vi "Get_ADAM_averages_server.vi"(5 "No of averages":i32=1, 6 "All Active Channels":bool, 7 "End time":dbl, 8 "Start time":dbl, 9 "Clients time":dbl, 10 "ADAM Ch Names":string[](array[string])) -> (0 "DBL values":dbl[][](array[numeric]) format="%.2f", 1 "Values":string[][](array[string]), 2 "Comments":string[](array[string]), 3 "Titles":string[](array[string]), 4 "Times":dbl[](array[numeric]) format="%.2f")   [LabVIEW 2021]
uses:
  ADAM_Global.vi
  Sub VI's/Logged_Data_real_Global.vi
  Sub VI's/Channel_Description_Global.vi
panel:
  out "Client leads me by:":dbl
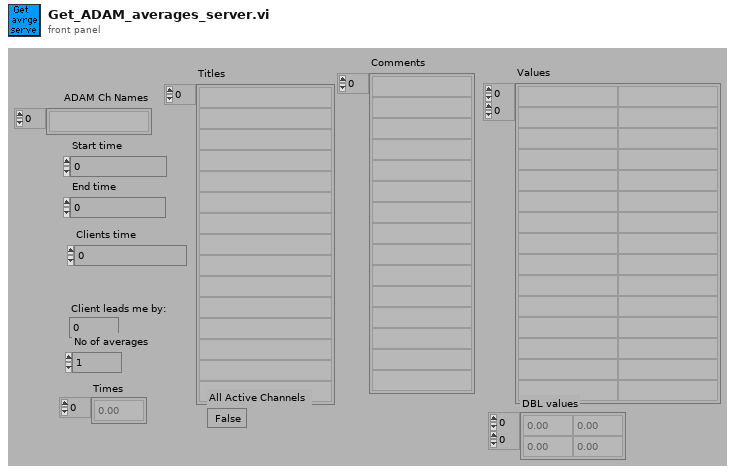
[diagram p1: front panel]
types:
  T1 = typedef "Update_scan_value.ctl" = cluster{"Channel Name":string, "New Value":dbl, "!Auto_Off":bool}
  T2 = typedef "Ch_description_ADAM.ctl" = cluster{"Ch Name":string, "Type":T3, "Function":T4, "Ch State":T5, "Calibration type":T6, "A":dbl, "B":dbl, "C":dbl, "D":dbl, "Comments":string, "Address":T7, "String":string, "Duty":u16}
  T3 = typedef "Module_type_ADAM.ctl" = string
  T4 = typedef "Function_ADAM.ctl" = enum16{"Analogue Input", "Digital Input", "Event counter", "Event rate", "Analogue Output", "Digital Output", "Relay Output"}
  T5 = typedef "Channel_State.ctl" = enum16{"On", "Off", "Always On", "Always Off"}
  T6 = typedef "Calib_type_ADAM.ctl" = string
  T7 = typedef "Address.ctl" = cluster{"Main":i32, "Ch.":i32, "Sub":i32, "Port Name":string}
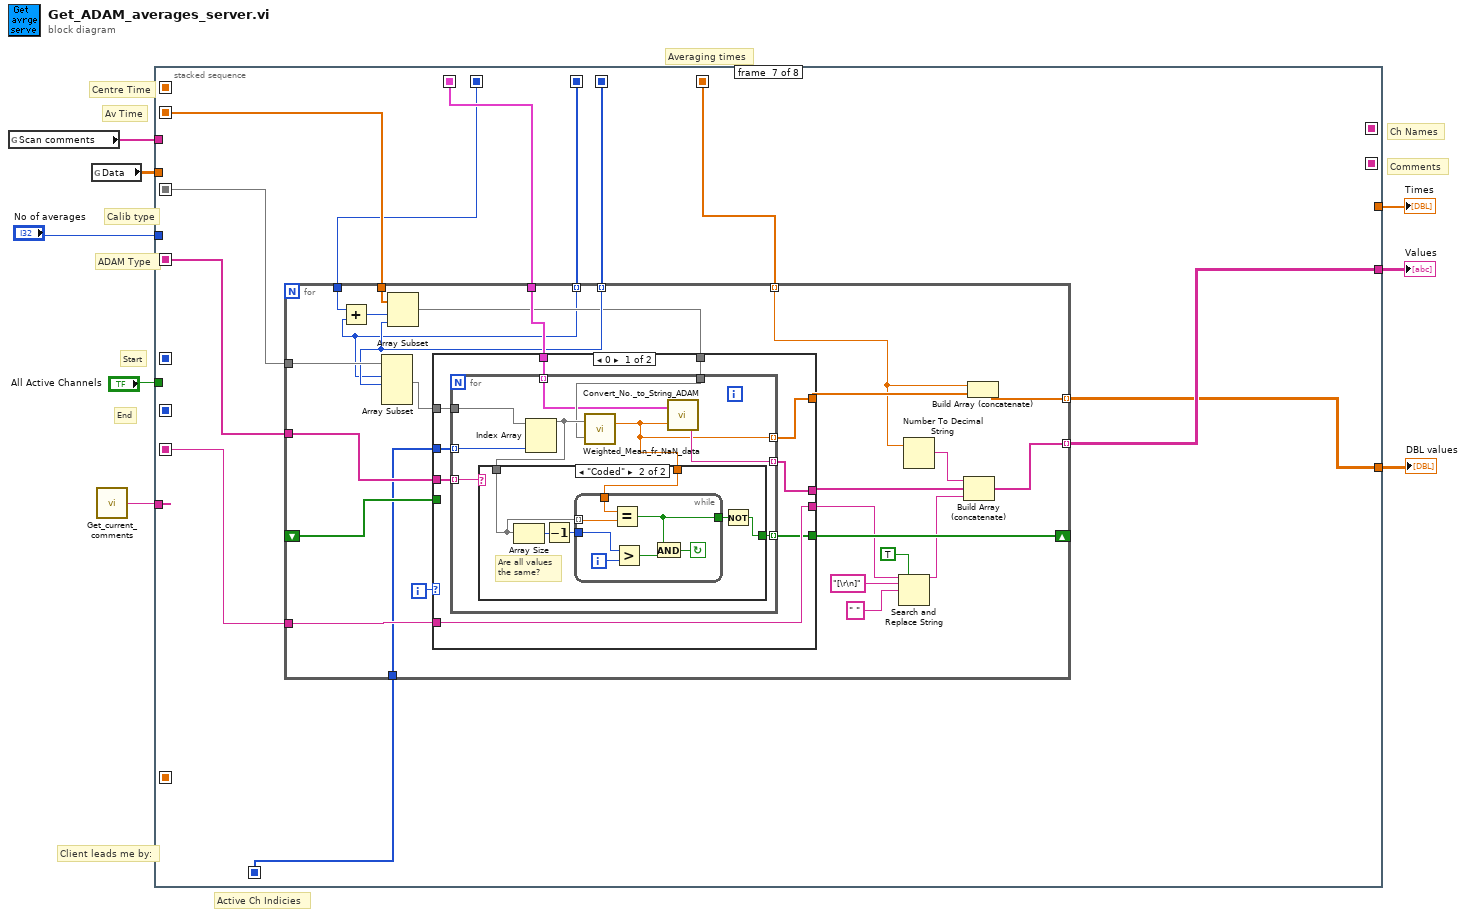
[diagram p0: block diagram]
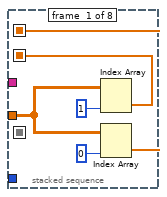
[diagram p2: hidden frame]
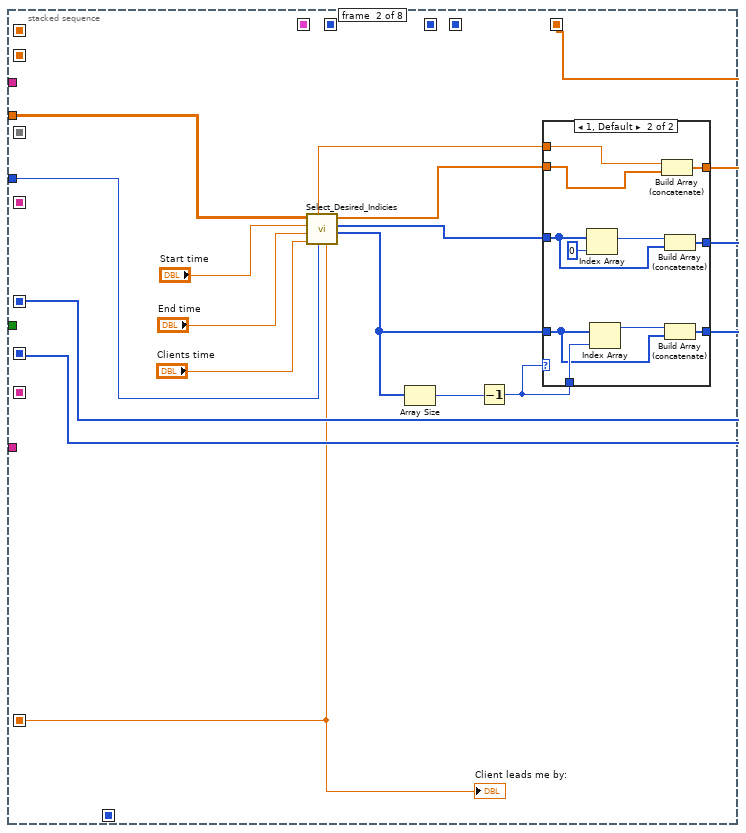
[diagram p3: hidden frame]
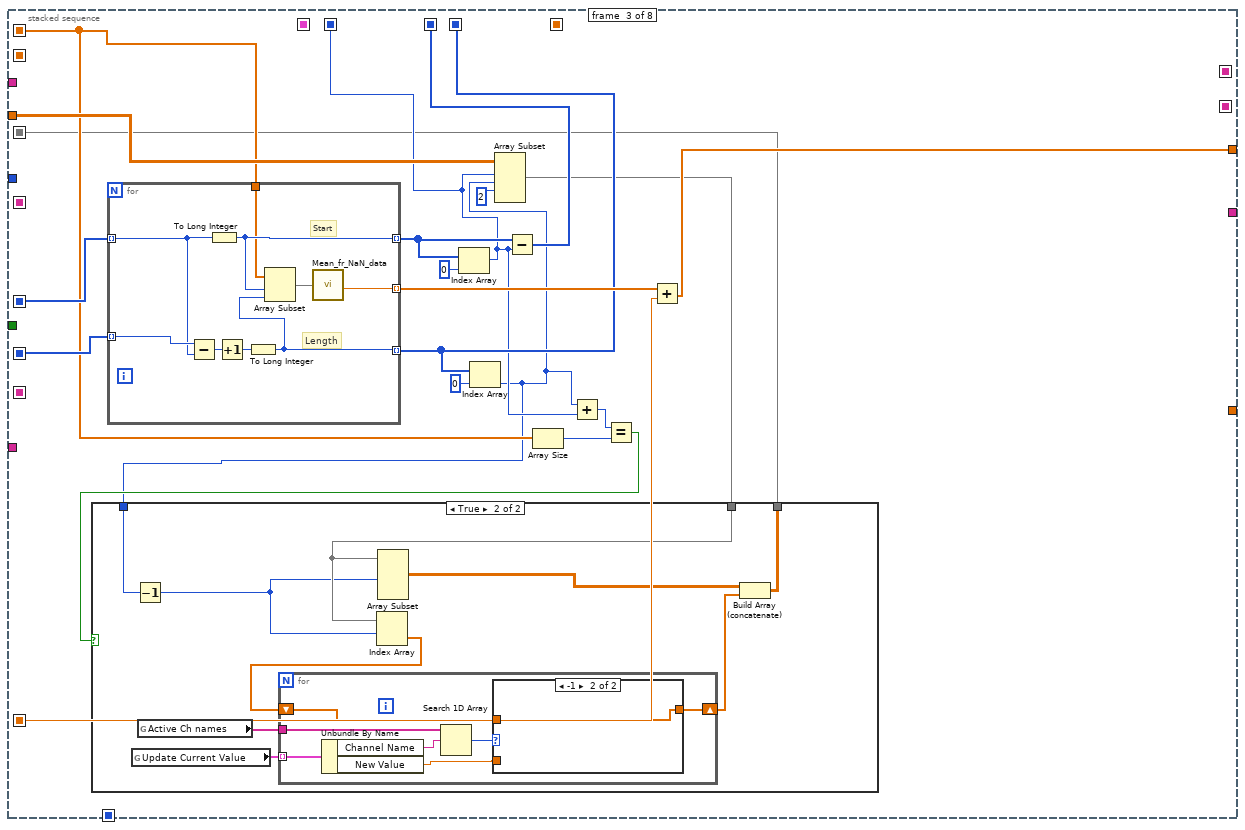
[diagram p5: hidden frame]
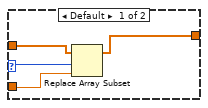
[diagram p7: hidden frame]
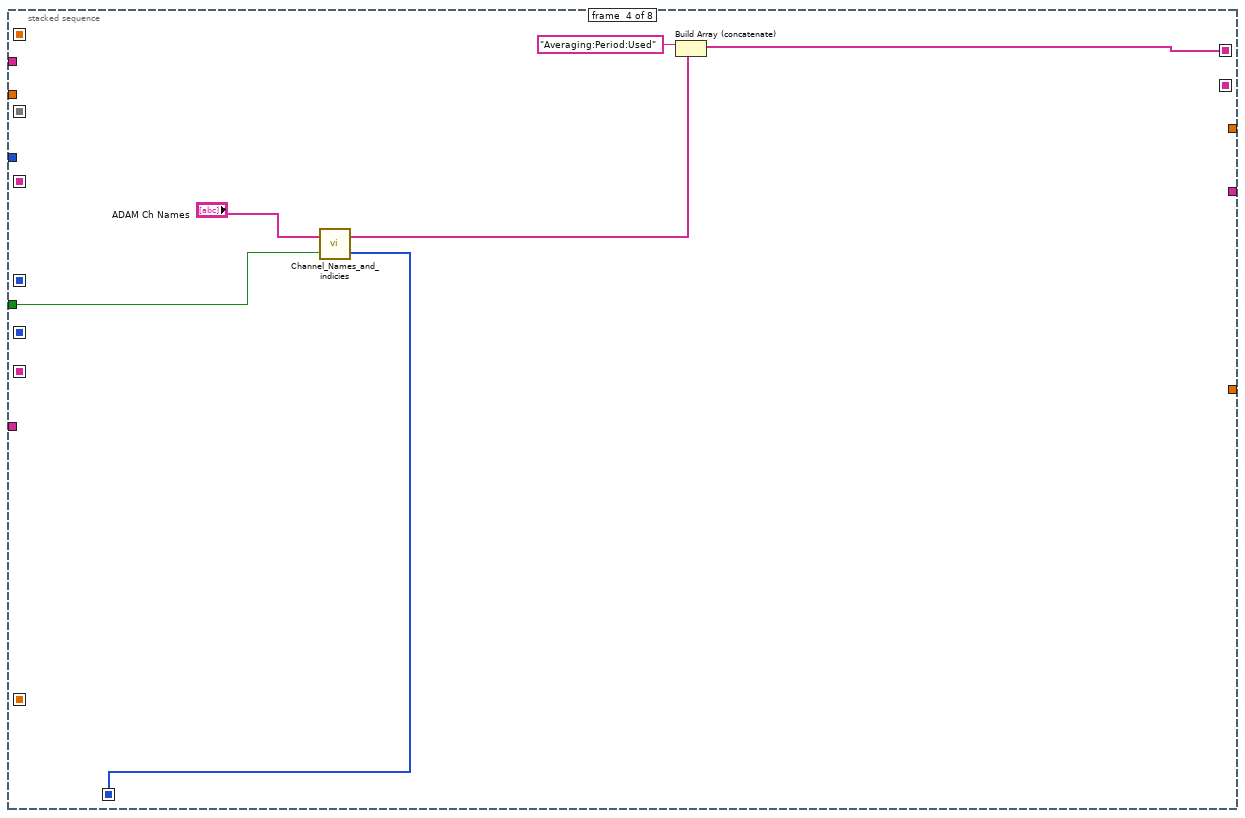
[diagram p8: hidden frame]
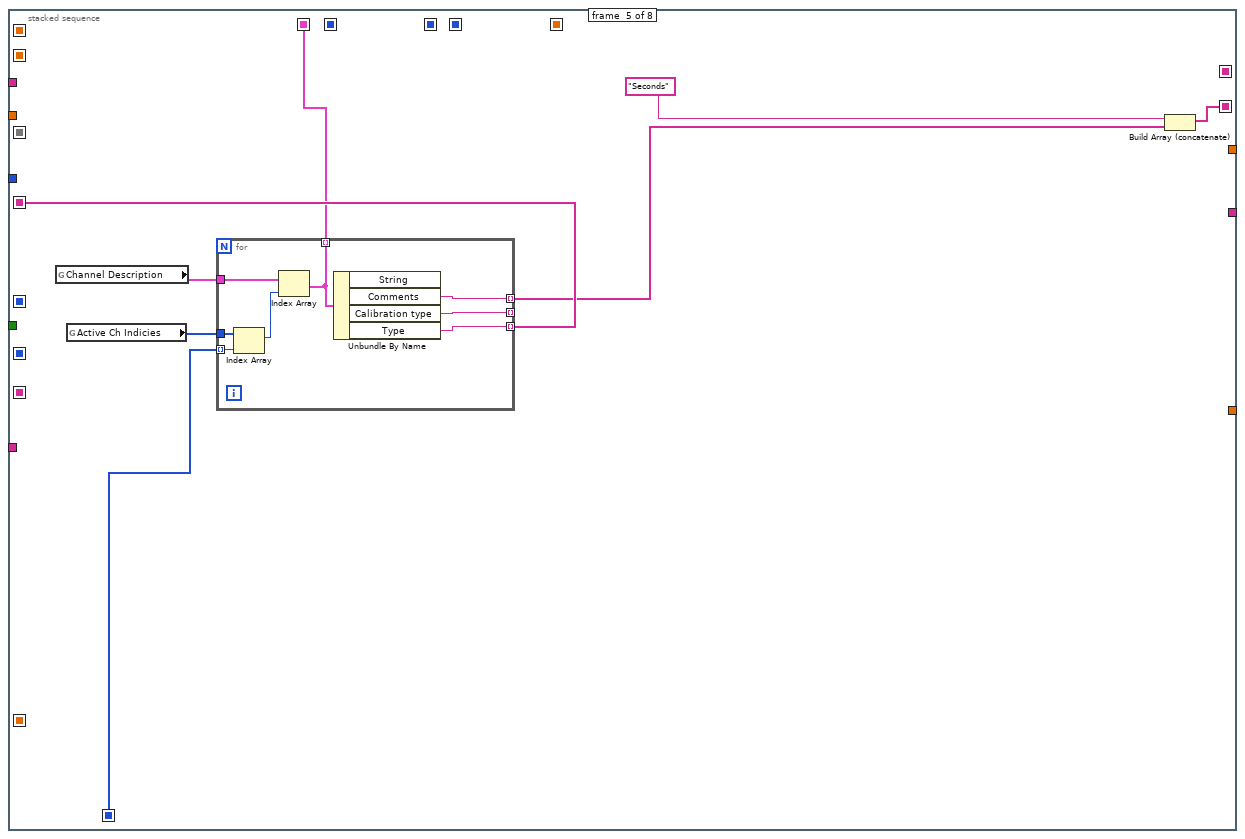
[diagram p9: hidden frame]
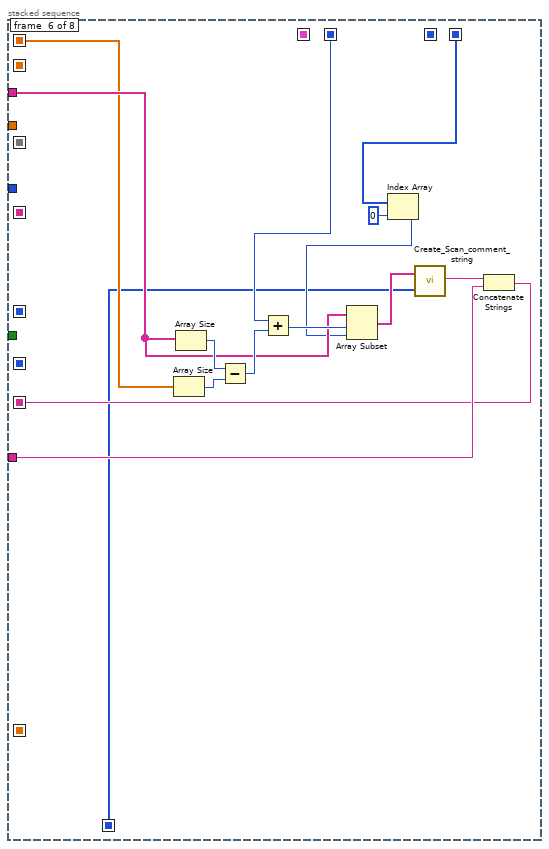
[diagram p10: hidden frame]
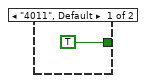
[diagram p11: hidden frame]
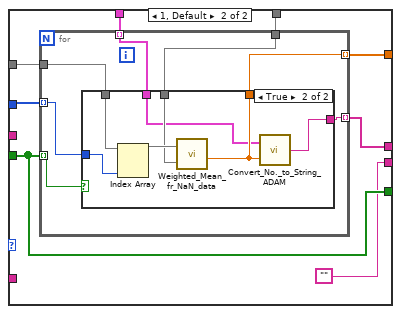
[diagram p12: hidden frame]
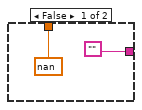
[diagram p13: hidden frame]
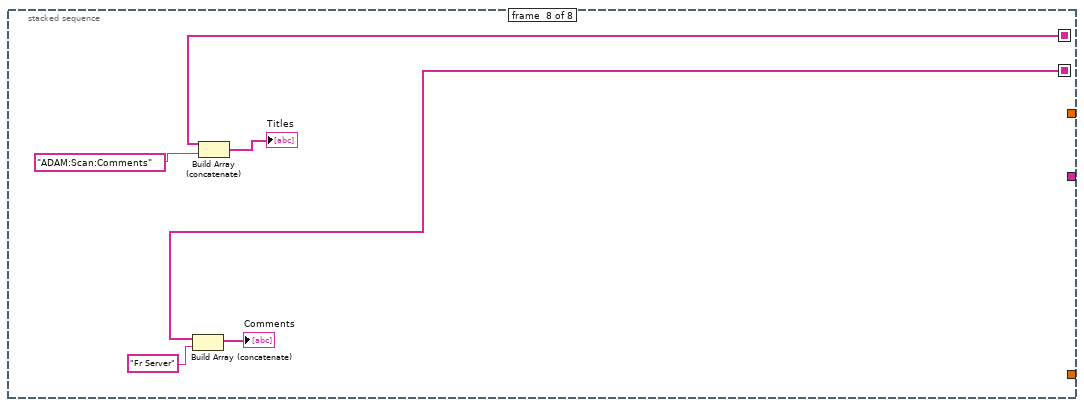
[diagram p14: hidden frame]
diagram:
  # "Averaging times"
  # "End"
  # "Start"
  # "Av Time"
  # "Centre Time"
  # "Active Ch Indicies"
  # "ADAM Type"
  # "Calib type"
  # "Ch Names"
  # "Comments"
  # "Client leads me by:"
  n1 = global read "ADAM_Global.vi" "Scan comments"() -> (w6:string[])
  n2 = global read "Logged_Data_real_Global.vi" "Data"() -> (w1:dbl[][])
  n3 = call "Get_current_comments.vi"() -> ("Comment"=w7:string)
  n4 = stacked-sequence {
    seq-local: [_ _ w54 _ _ _ _ _] -> [_ _ _ _ _ w121 w141 _]
    seq-local: [_ _ w56 _ _ _ _ _] -> [_ _ _ _ _ _ w142 _]
    seq-local: [_ _ w43 _ _ _ _ _] -> [_ _ _ _ _ _ w140 _]
    seq-local: [_ w28 _ _ _ _ _ _] -> [_ _ w60 _ _ _ _ _]
    seq-local: [_ w27 _ _ _ _ _ _] -> [_ _ w59 _ _ _ _ _]
    seq-local: [w11 _ _ _ _ _ _ _] -> [_ _ w49 _ _ w124 _ _]
    seq-local: [_ _ w50 _ _ _ _ _] -> [_ _ _ _ _ w123 w131 _]
    seq-local: [_ _ _ _ _ w117 _ _] -> [_ _ _ _ _ _ w138 _]
    seq-local: [_ _ _ _ w107 _ _ _] -> [_ _ _ _ _ _ w137 _]
    seq-local: [_ w14 _ _ _ _ _ _] -> [_ _ _ _ _ _ w136 _]
    seq-local: [_ _ _ w98 _ _ _ _] -> [_ _ _ _ _ _ _ w226]
    seq-local: [_ _ _ _ w104 _ _ _] -> [_ _ _ _ _ _ _ w225]
    seq-local: [_ w19 _ _ _ _ _ _] -> [_ _ w51 _ _ _ _ _]
    seq-local: [_ _ _ w95 _ _ _ _] -> [_ _ _ _ w102 w116 w134 _]
    seq-local: [w10 _ _ _ _ _ _ _] -> [_ _ _ _ _ _ w132 _]
    seq-local: [_ _ _ _ w100 _ _ _] -> [_ _ _ _ _ _ w133 _]
    tunnel: w1 -> [w9 w22 w53 _ _ _ _ _]
    tunnel: "No of averages" -> [_ w20 _ _ _ _ _ _]
    tunnel: [_ _ w61 _ _ _ _ _] -> w4
    tunnel: [_ _ _ _ _ _ w139 _] -> w5
    tunnel: [_ _ _ _ _ _ w135 _] -> w3
    tunnel: w6 -> [_ _ _ _ _ w125 _ _]
    tunnel: w7 -> [_ _ _ _ _ w118 _ _]
    tunnel: "All Active Channels" -> [_ _ _ w94 _ _ _ _]
    frame #0 {
      n5 = Index Array(array=w9, index (col)=1) -> (element=w10:dbl[])  [unwired: 1 in]
      n6 = Index Array(array=w9, index (col)=0) -> (element=w11:dbl[])  [unwired: 1 in]
    }
    frame #1 {
      n7 = call "Select_Desired_Indicies.vi"("No of averages"=w20, "Clients time"="Clients time", "End time"="End time", "Start time"="Start time", "Table values"=w22) -> ("End Integer"=w16:i32[], "Start integer"=w23:i32[], "Averaging Times"=w18:dbl[], "Client leads me by:"=w19:dbl, "Total Time"=w17:dbl)  [unwired: 1 out]
      "Client leads me by:" <- w19
      n8 = Array Size(array=w16) -> (size(s)=w15:i32)
      n9 = Decrement(x=w15) -> (x-1=w21:i32)
      n10 = case shown="1, Default" w21 {
        tunnel: w21 -> [_ w41]
        tunnel: w23 -> [w31 w39]
        tunnel: w16 -> [w30 w37]
        tunnel: [w31 w36] -> w28
        tunnel: [w30 w35] -> w27
        tunnel: [w29 w33] -> w14
        tunnel: w18 -> [w29 w34]
        tunnel: w17 -> [_ w32]
        frame 0 {
        }
        frame 1, Default {
          n11 = Index Array(array=w39, index=0 ("Index")) -> (element=w40:i32)
          n12 = Index Array(array=w37, index=w41) -> (element=w38:i32)
          n13 = Build Array (concatenate)(w32, w34) -> (w33:dbl[])
          n14 = Build Array (concatenate)(w40, w39) -> (w36:i32[])
          n15 = Build Array (concatenate)(w38, w37) -> (w35:i32[])
        }
      }
    }
    frame #2 {
      n16 = for {
        tunnel: [w91] -> w57 mode=indexing
        tunnel: [w85] -> w54 mode=indexing
        tunnel: [w89] -> w62 mode=indexing
        tunnel: w60 -> [w86] mode=indexing
        tunnel: w59 -> [w87] mode=indexing
        tunnel: w49 -> [w88]
        # "Length"
        # "Start"
        n17 = Subtract(x=w87, y=w86) -> (x-y=w92:i32)
        n18 = To Long Integer(number=w86) -> (32bit integer=w91:i32)
        n19 = Increment(x=w92) -> (x+1=w93:i32)
        n20 = To Long Integer(number=w93) -> (32bit integer=w85:i32)
        n21 = Array Subset(array=w88, index=w91, length=w85) -> (w90:dbl[])
        n22 = call "Mean_fr_NaN_data.vi"("Data"=w90) -> ("Mean value"=w89:dbl)  [unwired: 1 out]
      }
      n23 = Index Array(array=w57, index=0 ("Index")) -> (element=w50:i32)
      n24 = Index Array(array=w54, index=0 ("Index")) -> (element=w44:i32)
      n25 = Array Subset(array=w53, index (row)=w50, length (row)=w44, index (col)=2 ("Array Index")) -> (w45:dbl[][])  [unwired: 1 in]
      n26 = Subtract(x=w57, y=w50) -> (x-y=w56:i32[])
      n27 = Array Size(array=w49) -> (size(s)=w47:i32)
      n28 = Add(x=w44, y=w50) -> (x+y=w48:i32)
      n29 = Equal?(x=w48, y=w47) -> (x = y?=w46:bool)
      n30 = case shown="True" w46 {
        tunnel: w45 -> [w63 w70]
        tunnel: w44 -> [_ w72]
        tunnel: [w63 w66] -> w43
        frame False {
        }
        frame True {
          n31 = global read "ADAM_Global.vi" "Update Current Value"() -> (w68:T1[])
          n32 = Decrement(x=w72) -> (x-1=w69:i32)
          n33 = global read "ADAM_Global.vi" "Active Ch names"() -> (w67:string[])
          n34 = Index Array(array=w70, index (row)=w69) -> (element=w65:dbl[])  [unwired: 1 in]
          n35 = for {
            tunnel: w68 -> [w79] mode=indexing
            tunnel: w67 -> [w77]
            shift-right: [w73] -> w64
            shift-left: w65 -> [w74]
            n36 = Unbundle By Name(w79) -> ("Channel Name"=w78:string, "New Value"=w75:dbl)
            n37 = Search 1D Array(1D array=w77, element=w78) -> (index of element=w76:i32)  [unwired: 1 out]
            n38 = case shown="-1" w76 {
              selector: w76 -> [w80 _]
              tunnel: w75 -> [w83 _]
              tunnel: w74 -> [w82 w84]
              tunnel: [w81 w84] -> w73
              frame Default {
                n39 = Replace Array Subset(array=w82, new element=w83, index=w80) -> (w81:dbl[])
              }
              frame -1 {
              }
            }
          }
          n40 = Array Subset(array=w70, length (row)=w69) -> (w71:dbl[][])  [unwired: 3 in]
          n41 = Build Array (concatenate)(w71, w64) -> (w66:dbl[][])
        }
      }
      n42 = Add(x=w62, y=w51) -> (x+y=w61:dbl[])
    }
    frame #3 {
      n43 = call "Channel_Names_and_indicies.vi"("All Active Channels"=w94, "Desired Ch Names"="ADAM Ch Names") -> ("Indicies"=w95:i32[], "Active Ch names"=w96:string[])
      n44 = Build Array (concatenate)("Averaging:Period:Used" ("Input Element"), w96) -> (w98:string[])
    }
    frame #4 {
      n45 = global read "Channel_Description_Global.vi" "Channel Description"() -> (w101:T2[])
      n46 = global read "ADAM_Global.vi" "Active Ch Indicies"() -> (w103:i32[])
      n47 = for {
        tunnel: w101 -> [w115]
        tunnel: [w114] -> w105 mode=indexing
        tunnel: [w113] -> _ mode=indexing
        tunnel: [w112] -> w107 mode=indexing
        tunnel: w103 -> [w111]
        tunnel: w102 -> [w110] mode=indexing
        tunnel: [w108] -> w100 mode=indexing
        n48 = Index Array(array=w111, index=w110) -> (element=w109:i32)
        n49 = Index Array(array=w115, index=w109) -> (element=w108:T2)
        n50 = Unbundle By Name(w108) -> ("Comments"=w114:string, "Calibration type"=w113:T6, "Type"=w112:T3)  [unwired: 1 out]
      }
      n51 = Build Array (concatenate)("Seconds" ("Input Element"), w105) -> (w104:string[])
    }
    frame #5 {
      n52 = Array Size(array=w124) -> (size(s)=w128:i32)
      n53 = Array Size(array=w125) -> (size(s)=w127:i32)
      n54 = Subtract(x=w127, y=w128) -> (x-y=w129:i32)
      n55 = Add(x=w123, y=w129) -> (x+y=w130:i32)
      n56 = Index Array(array=w121, index=0 ("Index")) -> (element=w120:i32)
      n57 = Array Subset(array=w125, index=w130, length=w120) -> (w126:string[])
      n58 = call "Create_Scan_comment_string.vi"("Requested channels"=w116, "Scan comments"=w126) -> ("Comment string"=w119:string)
      n59 = Concatenate Strings(w119, w118) -> (w117:string)
    }
    frame #6 {
      n60 = for {
        tunnel: w142 -> [w149] mode=indexing
        tunnel: w141 -> [w152] mode=indexing
        tunnel: w140 -> [w168]
        tunnel: [w165] -> w139 mode=indexing
        tunnel: w138 -> [w162]
        tunnel: w137 -> [w164]
        shift-right: [w161] -> _
        shift-left: _ -> [w160]
        tunnel: w136 -> [w155] mode=indexing
        tunnel: w134 -> [w159]
        tunnel: [w156] -> w135 mode=indexing
        tunnel: w133 -> [w154]
        tunnel: w132 -> [w153]
        tunnel: w131 -> [w148]
        i -> [w163]
        n61 = Add(x=w148, y=w149) -> (x+y=w150:i32)
        n62 = Array Subset(array=w168, index (row)=w149, length (row)=w152) -> (w167:dbl[][])  [unwired: 2 in]
        n63 = Array Subset(array=w153, index=w150, length=w152) -> (w151:dbl[])
        n64 = case shown="0" w163 {
          tunnel: w167 -> [w177 w208]
          tunnel: [w176 w207] -> w166
          tunnel: w164 -> [w174 _]
          tunnel: w162 -> [w175 _]
          tunnel: [w175 ""] -> w144
          tunnel: [w173 w206] -> w161
          tunnel: w160 -> [_ w206]
          tunnel: w151 -> [w172 w204]
          tunnel: w159 -> [w171 w202]
          tunnel: [w170 w203] -> w157
          tunnel: w154 -> [w169 w201]
          frame 0 {
            n65 = for {
              tunnel: w177 -> [w185]
              tunnel: [w186] -> w176 mode=indexing
              tunnel: w174 -> [w184] mode=indexing
              tunnel: [w182] -> w173 mode=indexing
              tunnel: w172 -> [w181]
              tunnel: w171 -> [w180] mode=indexing
              tunnel: [w179] -> w170 mode=indexing
              tunnel: w169 -> [w178] mode=indexing
              n66 = Index Array(array=w185, index (col)=w180) -> (element=w183:dbl[])  [unwired: 1 in]
              n67 = call "Weighted_Mean_fr_NaN_data.vi"("Weighting"=w181, "Data"=w183) -> ("Mean value"=w179:dbl)
              n68 = case shown="\"Coded\"" w184 {
                tunnel: w183 -> [_ w191]
                tunnel: w179 -> [_ w190]
                tunnel: [TRUE w189] -> w182
                frame "4011", Default {
                }
                frame "Coded" {
                  # "Are all values the same?"
                  n69 = Array Size(array=w191) -> (size(s)=w192:i32)
                  n70 = Decrement(x=w192) -> (x-1=w193:i32)
                  n71 = while {
                    tunnel: w190 -> [w194]
                    tunnel: [w197] -> w188
                    tunnel: w191 -> [w196] mode=indexing
                    tunnel: w193 -> [w200]
                    i -> [w195]
                    stop <- w198 continue-if-true
                    n72 = Equal?(x=w194, y=w196) -> (x = y?=w197:bool)
                    n73 = Greater?(x=w200, y=w195) -> (0:w199:bool)
                    n74 = And(x=w197, y=w199) -> (x .and. y?=w198:bool)
                  }
                  n75 = Not(x=w188) -> (.not. x?=w189:bool)
                }
              }
              n76 = call "Convert_No._to_String_ADAM.vi"("Input number"=w179, "Ch Description"=w178) -> ("Output sting"=w186:string)
            }
          }
          frame 1, Default {
            n77 = for {
              tunnel: w208 -> [w214]
              tunnel: [w215] -> w207 mode=indexing
              tunnel: w206 -> [w213] mode=indexing
              tunnel: w204 -> [w212]
              tunnel: [w211] -> w203 mode=indexing
              tunnel: w202 -> [w210] mode=indexing
              tunnel: w201 -> [w209] mode=indexing
              n78 = case shown="True" w213 {
                tunnel: ["" w224] -> w215
                tunnel: w214 -> [_ w223]
                tunnel: w212 -> [_ w221]
                tunnel: [nan ("Mean value") w220] -> w211
                tunnel: w210 -> [_ w219]
                tunnel: w209 -> [_ w218]
                frame False {
                }
                frame True {
                  n79 = Index Array(array=w223, index (col)=w219) -> (element=w222:dbl[])  [unwired: 1 in]
                  n80 = call "Weighted_Mean_fr_NaN_data.vi"("Weighting"=w221, "Data"=w222) -> ("Mean value"=w220:dbl)
                  n81 = call "Convert_No._to_String_ADAM.vi"("Input number"=w220, "Ch Description"=w218) -> ("Output sting"=w224:string)
                }
              }
            }
          }
        }
        n82 = Search and Replace String(replace all?=TRUE ("replace all? (F)"), input string=w144, search string="[\r\n]" ("regular expression"), replace string=" " ("replace string (\"\")")) -> (result string=w143:string)  [unwired: 4 in, 3 out]
        n83 = Number To Decimal String(number=w155) -> (decimal integer string=w158:string)  [unwired: 1 out]
        n84 = Build Array (concatenate)(w158, w166, w143) -> (w165:string[])
        n85 = Build Array (concatenate)(w155, w157) -> (w156:dbl[])
      }
    }
    frame #7 {
      n86 = Build Array (concatenate)(w225, "Fr Server" ("Comments")) -> (→"Comments":string[])
      n87 = Build Array (concatenate)(w226, "ADAM:Scan:Comments") -> (→"Titles":string[])
    }
  }
  "Values" <- w5
  "Times" <- w4
  "DBL values" <- w3
